vi "Elevator Sensor Tasks.vi"(0 "SecondUpperElevatorSwitchDevRef":T1={"DevStatus"={"status"=FALSE, "code"=0, "source"=""}, "DIO Channel"=enum."Invalid", "CntIndex"=enum."Invalid", "Normally Closed"=FALSE}, 1 "SecondLowerElevatorSwitchDevRef":T1={"DevStatus"={"status"=FALSE, "code"=0, "source"=""}, "DIO Channel"=enum."Invalid", "CntIndex"=enum."Invalid", "Normally Closed"=FALSE}, 2 "ElevatorControllerDevRef":T4={"DeviceStatus"={"status"=FALSE, "code"=0, "source"=""}, "Type"=enum."PWM", "PWM"={"PWM Channel"=enum."Invalid", "DeadBand"={"Name"="", "maxPositivePwm"=0, "minPositivePwm"=0, "centerPwm"=0, "maxNegativePwm"=0, "minNegativePwm"=0, "angularRange"=0}}, "CAN"={"Device Number"=0, "SetOutput VI Ref"=variant(refnum<vi> refnum), "GetOutput VI Ref"=variant(refnum<vi> refnum), "Enable VI Ref"=variant(refnum<vi> refnum), "Disable VI Ref"=variant(refnum<vi> refnum), "Data"=variant}, "Invert"=FALSE, "DIO PWM"={"PWM \"Enable\" Channel"=enum."Invalid", "DIOChannel"=enum."Invalid", "PWM Rate"=0.0}}, 3 "FirstLowerElevatorSwitchDevRef":T1={"DevStatus"={"status"=FALSE, "code"=0, "source"=""}, "DIO Channel"=enum."Invalid", "CntIndex"=enum."Invalid", "Normally Closed"=FALSE}) -> ()   [LabVIEW 2017]
uses:
  <vilib>/Rock Robotics/WPI/MotorControl/WPI_MotorControlDeviceRef.ctl
  <vilib>/Rock Robotics/WPI/MotorControl/WPI_MotorControlType.ctl
  <vilib>/Rock Robotics/SystemInterfaces/DIO/FPGA_DIOPWMChannel.ctl
  <vilib>/Rock Robotics/WPI/PWM/WPI_PWMDeadband.ctl
  <vilib>/Rock Robotics/SystemInterfaces/DIO/FPGA_DIOChannel.ctl
  <vilib>/Rock Robotics/WPI/Switch/WPI_SwitchDevRef.ctl
  <vilib>/Rock Robotics/SystemInterfaces/Counter/FPGA_CounterCtrSystemIndex.ctl
  Implementation/Elevator Published Globals.vi
  <vilib>/Rock Robotics/WPI/ThirdParty/Phoenix-LabVIEW/Motor Controller/Get/CTRE_Phoenix_MotorController_GetSelectedSensorData.vi
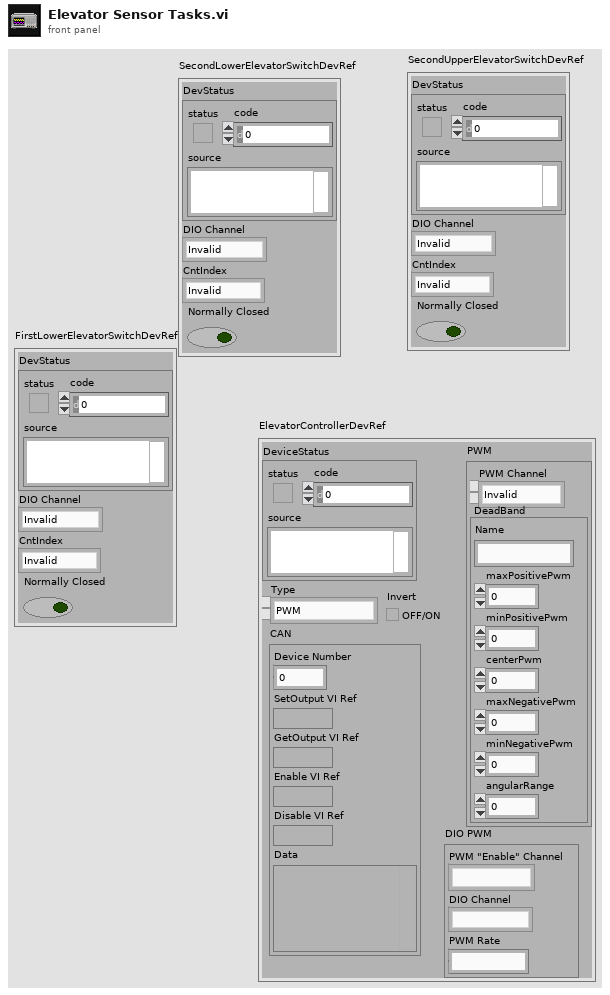
[diagram p1: front panel]
types:
  T1 = typedef "WPI_SwitchDevRef.ctl" = cluster{"DevStatus":errorcluster, "DIO Channel":T2, "CntIndex":T3, "Normally Closed":bool}
  T2 = typedef "FPGA_DIOChannel.ctl" = enum8{"DIO 0", "DIO 1", "DIO 2", "DIO 3", "DIO 4", "DIO 5", "DIO 6", "DIO 7", "DIO 8", "DIO 9", "DIO MXP 0", "DIO MXP 1", "DIO MXP 2", "DIO MXP 3", "DIO MXP 4", "DIO MXP 5", "DIO MXP 6", "DIO MXP 7", "DIO MXP 8", "DIO MXP 9", "DIO MXP 10", "DIO MXP 11", "DIO MXP 12", "DIO MXP 13", "DIO MXP 14", "DIO MXP 15", "SPI Port CS1", "SPI Port CS2", "SPI Port CS3", "SPI Port MISO", "SPI Port MOSI", "Invalid"}
  T3 = typedef "FPGA_CounterCtrSystemIndex.ctl" = enum8{"Ctr 0", "Ctr 1", "Ctr 2", "Ctr 3", "Ctr 4", "Ctr 5", "Ctr 6", "Ctr 7", "Invalid"}
  T4 = typedef "WPI_MotorControlDeviceRef.ctl" = cluster{"DeviceStatus":errorcluster, "Type":T5, "PWM":cluster{"PWM Channel":T6, "DeadBand":T7}, "CAN":cluster{"Device Number":u8, "SetOutput VI Ref":variant, "GetOutput VI Ref":variant, "Enable VI Ref":variant, "Disable VI Ref":variant, "Data":variant}, "Invert":bool, "DIO PWM":cluster{"PWM \"Enable\" Channel":T6, "DIOChannel":T2, "PWM Rate":dbl}}
  T5 = typedef "WPI_MotorControlType.ctl" = enum16{"PWM", "CAN", "DIO PWM"}
  T6 = typedef "FPGA_DIOPWMChannel.ctl" = enum8{"PWM 0", "PWM 1", "PWM 2", "PWM 3", "PWM 4", "PWM 5", "PWM 6", "PWM 7", "PWM 8", "PWM 9", "PWM MXP 0", "PWM MXP 1", "PWM MXP 2", "PWM MXP 3", "PWM MXP 4", "PWM MXP 5", "PWM MXP 6", "PWM MXP 7", "PWM MXP 8", "PWM MXP 9", "Invalid"}
  T7 = typedef "WPI_PWMDeadband.ctl" = cluster{"Name":string, "maxPositivePwm":i32, "minPositivePwm":i32, "centerPwm":i32, "maxNegativePwm":i32, "minNegativePwm":i32, "angularRange":u16}
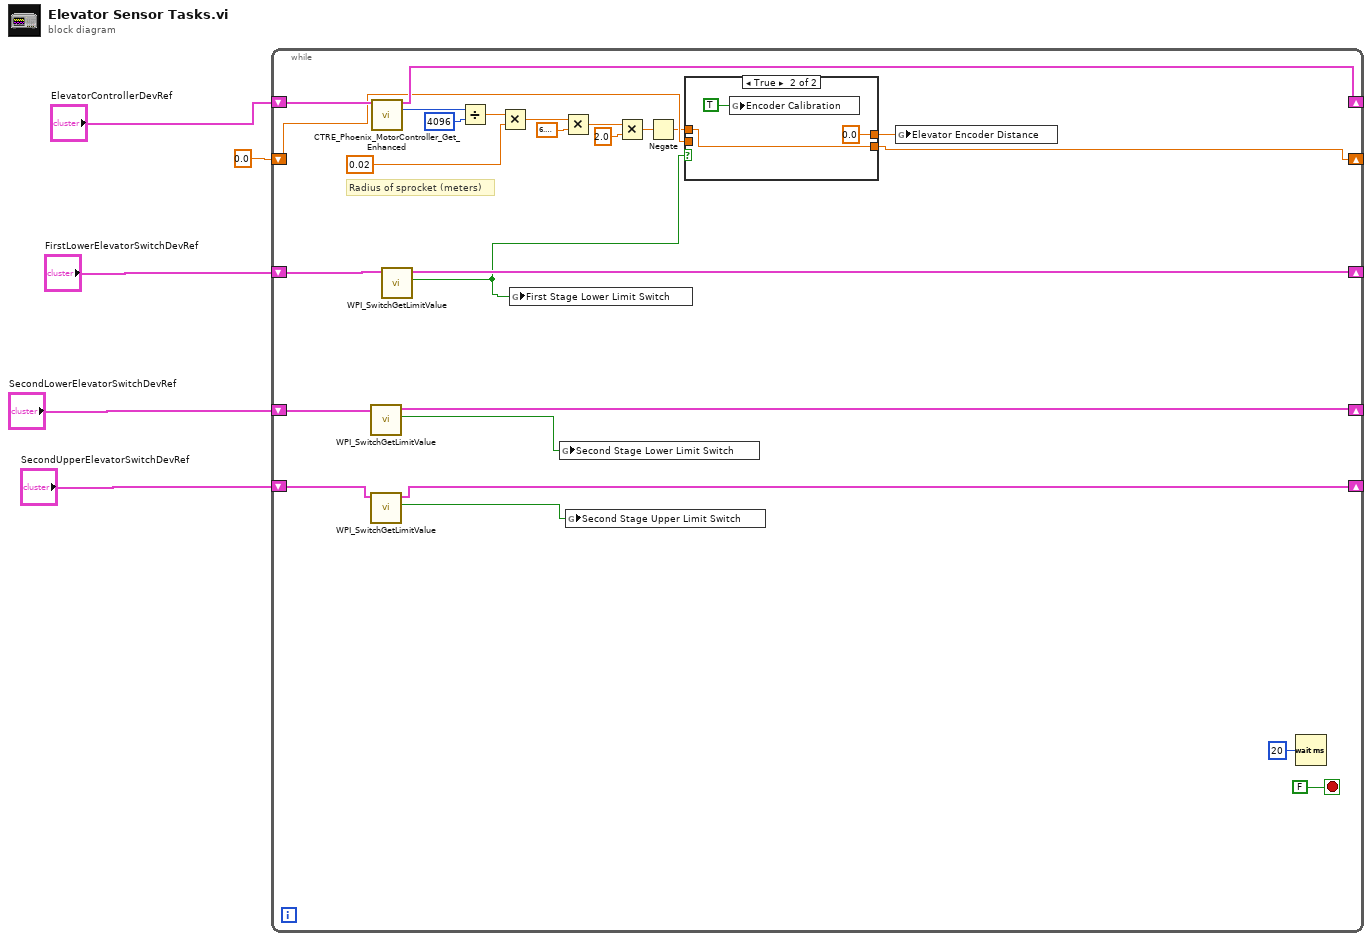
[diagram p0: block diagram]
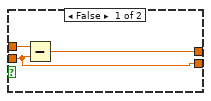
[diagram p2: hidden frame]
diagram:
  n1 = while {
    shift-right: [w29] -> _
    shift-left: "ElevatorControllerDevRef" -> [w28]
    shift-right: [w23] -> _
    shift-left: "FirstLowerElevatorSwitchDevRef" -> [w24]
    shift-right: [w18] -> _
    shift-left: "SecondUpperElevatorSwitchDevRef" -> [w20]
    shift-right: [w19] -> _
    shift-left: "SecondLowerElevatorSwitchDevRef" -> [w21]
    shift-right: [w14] -> _
    shift-left: 0.0 -> [w12]
    stop <- FALSE stop-if-true
    # "Radius of sprocket (meters)"
    n2 = call <vilib>:"WPI_SwitchGetLimitValue.vi"("SwitchDevRef"=w21) -> ("Switch Pressed"=w17:bool, "SwitchDevRef"=w19:T1)  [unwired: 8 in, 1 out]
    n3 = call <vilib>:"WPI_SwitchGetLimitValue.vi"("SwitchDevRef"=w20) -> ("Switch Pressed"=w16:bool, "SwitchDevRef"=w18:T1)  [unwired: 8 in, 1 out]
    n4 = call-poly <vilib>:"CTRE_Phoenix_MotorController_Get_Enhanced.vi"("PhoenixMotorControlDevRef"=w28) -> ("PhoenixMotorControlDevRef"=w29:T4, "Position (Raw Sensor Units)"=w31:i32)  [unwired: 11 in, 2 out]
    n5 = call <vilib>:"WPI_SwitchGetLimitValue.vi"("SwitchDevRef"=w24) -> ("Switch Pressed"=w15:bool, "SwitchDevRef"=w23:T1)  [unwired: 8 in, 1 out]
    n6 = Divide(x=w31, y=4096) -> (x/y=w27:dbl)
    n7 = Multiply(x=w27, y=0.02) -> (x*y=w10:dbl)
    n8 = global write "Elevator Published Globals.vi" "First Stage Lower Limit Switch"(w15) -> ()
    n9 = global write "Elevator Published Globals.vi" "Second Stage Lower Limit Switch"(w17) -> ()
    n10 = Multiply(x=w10, y=6.283185307179586) -> (x*y=w8:dbl)
    n11 = global write "Elevator Published Globals.vi" "Second Stage Upper Limit Switch"(w16) -> ()
    n12 = Multiply(x=w8, y=2.0) -> (x*y=w6:dbl)
    n13 = Negate(x=w6) -> (-x=w11:dbl)
    n14 = case shown="True" w15 {
      tunnel: w11 -> [w34 w37]
      tunnel: [w32 w37] -> w14
      tunnel: [w33 0.0] -> w13
      tunnel: w12 -> [w32 _]
      frame False {
        n15 = Subtract(x=w34, y=w32) -> (x-y=w33:dbl)
      }
      frame True {
        n16 = global write "Elevator Published Globals.vi" "Encoder Calibration"(TRUE) -> ()
      }
    }
    n17 = global write "Elevator Published Globals.vi" "Elevator Encoder Distance"(w13) -> ()
    n18 = Wait (ms)(milliseconds to wait=u32 20) -> ()  [unwired: 1 out]
  }
